vi "Choose Sphere.vi"(8 "error in (no error)":errorcluster, 11 "Hardware Configuration In":T1) -> (0 "error out":errorcluster, 2 "Sphere Indicator":T3, 3 "Hardware Configuration Out":T1)   [LabVIEW 2013]
uses:
  Hardware Configuration.ctl
  Libraries/AS-5216-DLL/AVS settings.ctl
  Sphere Indicator.ctl
  AvaSpec Acquisition.lvlib
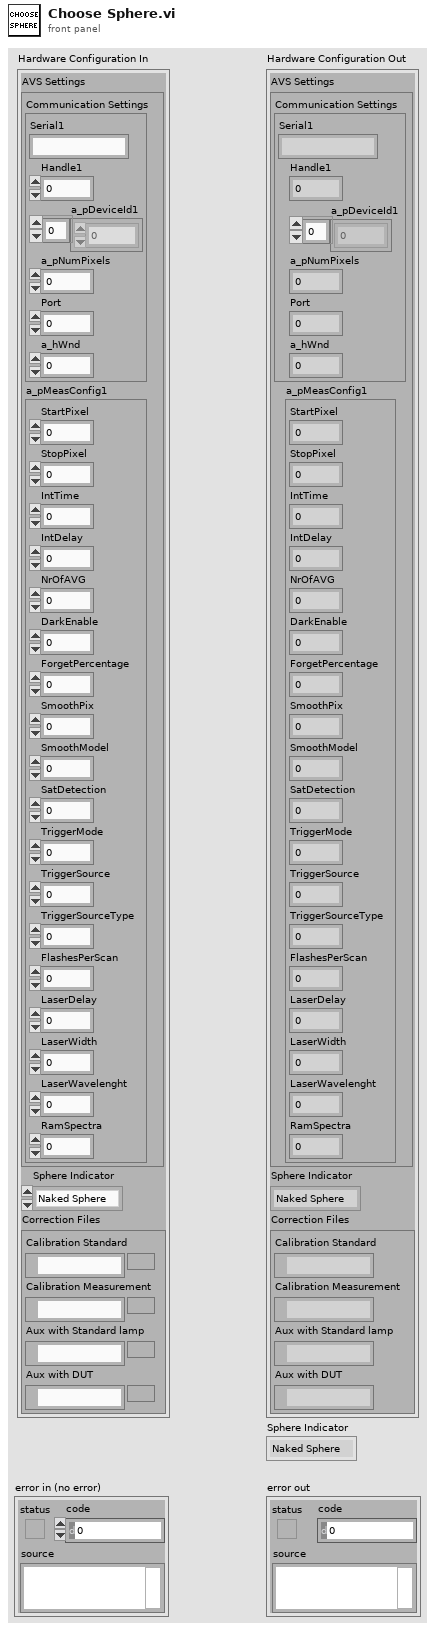
[diagram p1: front panel]
types:
  T1 = typedef "AvaSpec Acquisition.lvlib/Hardware Configuration.ctl" = cluster{"AVS Settings":T2, "Sphere Indicator":T3, "Correction Files":cluster{"Calibration Standard":path, "Calibration Measurement":path, "Aux with DUT":path, "Aux with Standard lamp":path}}
  T2 = typedef "AVS settings.ctl" = cluster{"Communication Settings":cluster{"Serial1":string, "Handle1":i32, "a_pDeviceId1":u8[], "a_pNumPixels":u16, "Port":i32, "a_hWnd":i32}, "a_pMeasConfig1":cluster{"StartPixel":u16, "StopPixel":u16, "IntTime":sgl, "IntDelay":u32, "NrOfAVG":u32, "DarkEnable":u8, "ForgetPercentage":u8, "SmoothPix":u16, "SmoothModel":u8, "SatDetection":u8, "TriggerMode":u8, "TriggerSource":u8, "TriggerSourceType":u8, "FlashesPerScan":u16, "LaserDelay":u32, "LaserWidth":u32, "LaserWavelenght":sgl, "RamSpectra":u16}}
  T3 = typedef "Sphere Indicator.ctl" = enum16{"Naked Sphere", "Insulated Sphere"}
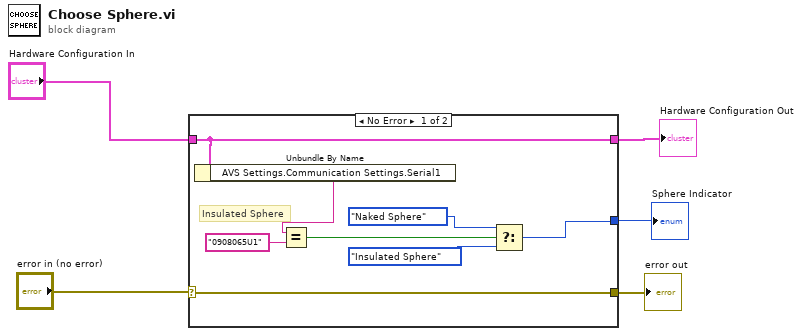
[diagram p0: block diagram]
diagram:
  n1 = case shown="No Error" "error in (no error)" {
    selector: "error in (no error)" -> [w13 w14]
    tunnel: [w13 w14] -> w4
    tunnel: "Hardware Configuration In" -> [w12 w15]
    tunnel: [w12 w15] -> w2
    tunnel: [w6 _] -> w1
    frame No Error {
      # "Insulated Sphere"
      n2 = Unbundle By Name(w12) -> ("AVS Settings.Communication Settings.Serial1"=w11:string)
      n3 = Equal?(x=w11, y="0908065U1") -> (x = y?=w9:bool)
      n4 = Select(t=Sphere_Indicator."Naked Sphere", s=w9, f=Sphere_Indicator."Insulated Sphere") -> (s? t:f=w6:T3)
    }
    frame Error {
    }
  }
  "error out" <- w4
  "Hardware Configuration Out" <- w2
  "Sphere Indicator" <- w1
